vi "test_CRIO daqmx PWM Open Collector.vi"() -> ()   [LabVIEW 2023]
uses:
  DIO/Virtual DIO/Virt PWM Generator/Virt DAQmx PWM Generator.lvclass
  <vilib>/DAQmx/write.llb/DAQmx Write (Digital 1D U32 1Chan NSamp).vi
  <vilib>/DAQmx/create/channels.llb/DAQmx Create Channel (DO-Digital Output).vi
  <vilib>/DAQmx/configure/timing.llb/DAQmx Timing (Sample Clock).vi
  <vilib>/DAQmx/miscellaneous.llb/DAQmx Fill In Error Info.vi
panel:
  out "Waveform Graph":u16[](graph)
  in  "Duty Cycle":dbl=10.0 caption="Duty Cycle (%)" format="%#_g %"
  out "error out":errorcluster
  in  "Stop":bool
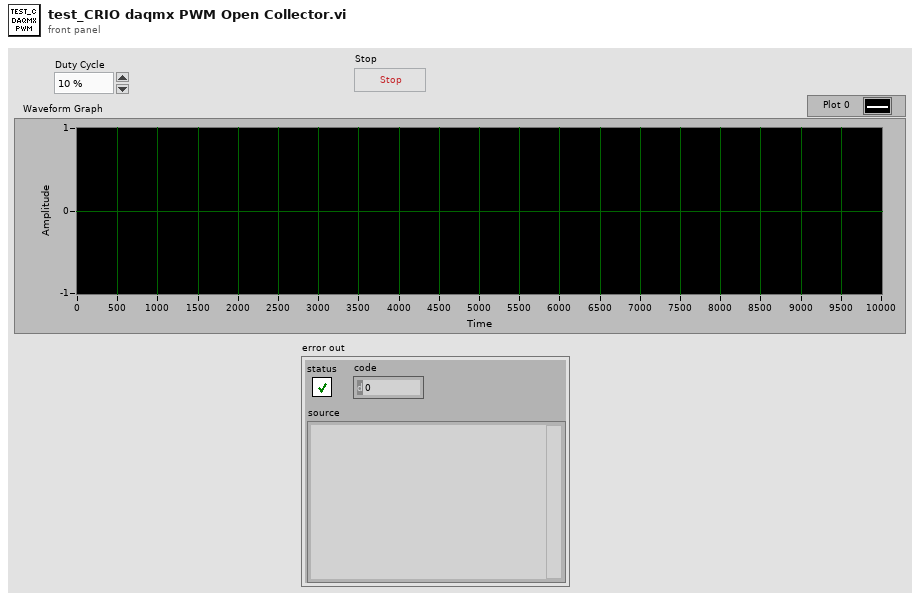
[diagram p1: front panel]
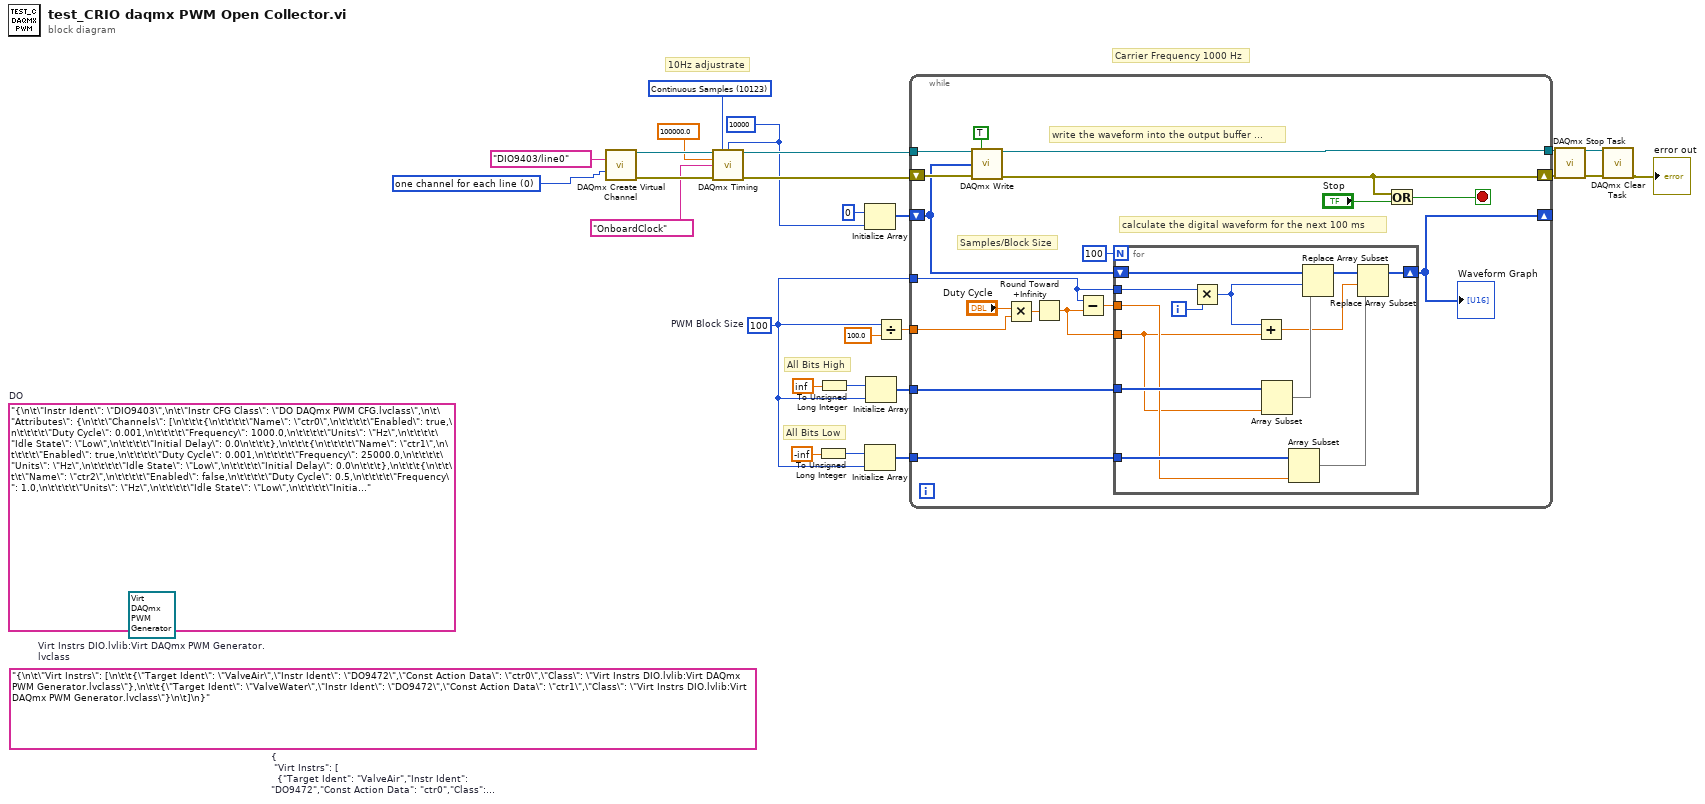
[diagram p0: block diagram]
diagram:
  w1 = 0 items=["one channel for each line", "one channel for all lines"] ("line grouping")
  w2 = 100  # PWM Block Size
  w12 = 10000
  w15 = 10123 items=["Finite Samples"=10178, "Continuous Samples"=10123, "Hardware Timed Single Point"=12522] ("sample mode")
  (unwired) refnum<class "Virt DAQmx PWM Generator.lvclass"> refnum  # Virt Instrs DIO.lvlib:Virt DAQmx PWM Generator.lvclass
  (unwired) "{\n\t\"Instr Ident\": \"DIO9403\",\n\t\"Instr CFG Class\": \"DO DAQmx PWM CFG.lvclass\",\n\t\"Attributes\": {\n\t\t\"Channels\": [\n\t\t\t{\n\t\t\t\t\"Name\": \"ctr0\",\n\t\t\t\t\"Enabled\": true,\n\t\t\t\t\"Duty Cycle\": 0.001,\n\t\t\t\t\"Frequency\": 1000.0,\n\t\t\t\t\"Units\": \"Hz\",\n\t\t\t\t\"Idle State\": \"Low\",\n\t\t\t\t\"Initial Delay\": 0.0\n\t\t\t},\n\t\t\t{\n\t\t\t\t\"Name\": \"ctr1\",\n\t\t\t\t\"Enabled\": true,\n\t\t\t\t\"Duty Cycle\": 0.001,\n\t\t\t\t\"Frequency\": 25000.0,\n\t\t\t\t\"Units\": \"Hz\",\n\t\t\t\t\"Idle State\": \"Low\",\n\t\t\t\t\"Initial Delay\": 0.0\n\t\t\t},\n\t\t\t{\n\t\t\t\t\"Name\": \"ctr2\",\n\t\t\t\t\"Enabled\": false,\n\t\t\t\t\"Duty Cycle\": 0.5,\n\t\t\t\t\"Frequency\": 1.0,\n\t\t\t\t\"Units\": \"Hz\",\n\t\t\t\t\"Idle State\": \"Low\",\n\t\t\t\t\"Initial Delay\": 0.0\n\t\t\t},\n\t\t\t{\n\t\t\t\t\"Name\": \"ctr3\",\n\t\t\t\t\"Enabled\": false,\n\t\t\t\t\"Duty Cycle\": 0.5,\n\t\t\t\t\"Frequency\": 1.0,\n\t\t\t\t\"Units\": \"Hz\",\n\t\t\t\t\"Idle State\": \"Low\",\n\t\t\t\t\"Initial Delay\": 0.0\n\t\t\t}\n\t\t],\n\t\t\"Timing\": {\n\t\t\t\"Samples per Channel\": 1000,\n\t\t\t\"Sample Mode\": \"Continuous Samples\",\n\t\t\t\"Sample Rate\": 0.0,\n\t\t\t\"Sample Clock Source\": \"Implicit\",\n\t\t\t\"Active Edge\": \"Rising\"\n\t\t},\n\t\t\"Trigger\": {\n\t\t\t\"Trigger Type\": \"No Trigger\"\n\t\t}\n\t}\n}"  # DO
  (unwired) "{\n\t\"Virt Instrs\": [\n\t\t{\"Target Ident\": \"ValveAir\",\"Instr Ident\": \"DO9472\",\"Const Action Data\": \"ctr0\",\"Class\": \"Virt Instrs DIO.lvlib:Virt DAQmx PWM Generator.lvclass\"},\n\t\t{\"Target Ident\": \"ValveWater\",\"Instr Ident\": \"DO9472\",\"Const Action Data\": \"ctr1\",\"Class\": \"Virt Instrs DIO.lvlib:Virt DAQmx PWM Generator.lvclass\"}\n\t]\n}"  # { 	"Virt Instrs": [ 		{"Target Ident": "ValveAir","Instr Ident": "DO9472","Const Action Data": "ctr0","Class": "Virt Instrs DIO.lvlib:Virt DAQmx PWM Generator.lvclass"}, 		{"Target Ident": "ValveWater","Instr Ident": "DO9472","Const Action Data": "ctr1","Class": "Virt Instrs DIO.lvlib:Virt DAQmx PWM Generator.lvclass"} 	] }
  # "Carrier Frequency 1000 Hz"
  # "All Bits Low"
  # "All Bits High"
  # "10Hz adjustrate"
  n1 = call-poly <vilib>:"DAQmx Create Virtual Channel.vi"("lines"=tag "DIO9403/line0", "line grouping"=w1) -> ("task out"=w18:refnum<k21>, "error out"=w20:errorcluster)  [unwired: 12 in]
  n2 = call-poly <vilib>:"DAQmx Timing.vi"("task/channels in"=w18, "sample mode"=w15, "samples per channel"=w12, "rate"=100000.0, "source"=tag "OnboardClock", "error in"=w20) -> ("task out"=w17:refnum<k21>, "error out"=w19:errorcluster)  [unwired: 8 in]
  n3 = To Unsigned Long Integer(number=-inf) -> (unsigned 32bit integer=w8:u32)
  n4 = To Unsigned Long Integer(number=inf) -> (unsigned 32bit integer=w9:u32)
  n5 = Initialize Array(u16 0 ("element"), w12) -> (w13:u16[])
  n6 = Initialize Array(w8, w2) -> (w6:u32[])
  n7 = Initialize Array(w9, w2) -> (w5:u32[])
  n8 = Divide(x=w2, y=100.0) -> (x/y=w3:dbl)
  n9 = while {
    tunnel: w17 -> [w43]
    shift-right: [w41] -> w22
    shift-left: w19 -> [w44]
    tunnel: [w42] -> w23
    shift-right: [w27] -> _
    shift-left: w13 -> [w29]
    tunnel: w6 -> [w32]
    tunnel: w5 -> [w31]
    tunnel: w3 -> [w36]
    tunnel: w2 -> [w28]
    stop <- w40 stop-if-true
    # "Samples/Block Size"
    # "calculate the digital waveform for the next 100 ms"
    # "write the waveform into the output buffer ..."
    n10 = call-poly <vilib>:"DAQmx Write.vi"("task/channels in"=w43, "auto start"=TRUE, "data"=w29, "error in"=w44) -> ("task out"=w42:refnum<k21>, "error out"=w41:errorcluster)  [unwired: 9 in, 1 out]
    n11 = Multiply(x="Duty Cycle", y=w36) -> (x*y=w35:dbl)
    n12 = Round Toward +Infinity(x=w35) -> (ceil(x): smallest int >= x=w30:dbl)
    n13 = Subtract(x=w28, y=w30) -> (x-y=w33:dbl)
    n14 = for {
      N: 100 -> [_]
      shift-right: [w57] -> w27
      shift-left: w29 -> [w56]
      tunnel: w33 -> [w50]
      tunnel: w30 -> [w46]
      tunnel: w31 -> [w54]
      tunnel: w32 -> [w53]
      tunnel: w28 -> [w49]
      i -> [w48]
      n15 = Multiply(x=w49, y=w48) -> (x*y=w47:i32)
      n16 = Add(x=w47, y=w46) -> (x+y=w45:dbl)
      n17 = Array Subset(array=w54, length=w46) -> (w51:u32[])  [unwired: 1 in]
      n18 = Array Subset(array=w53, length=w50) -> (w52:u32[])  [unwired: 1 in]
      n19 = Replace Array Subset(array=w56, new element=w51, index=w47) -> (w55:u16[])
      n20 = Replace Array Subset(array=w55, new element=w52, index=w45) -> (w57:u16[])
    }
    "Waveform Graph" <- w27
    n21 = Or(x=w41, y="Stop") -> (x .or. y?=w40:bool)
  }
  n22 = call <vilib>:"DAQmx Stop Task.vi"("task/channels in"=w23, "error in"=w22) -> ("task out"=w24:refnum<k21>, "error out"=w25:errorcluster)  [unwired: 12 in]
  n23 = call <vilib>:"DAQmx Clear Task.vi"("task in"=w24, "error in"=w25) -> ("error out"=→"error out":errorcluster)  [unwired: 13 in]
